vi "Close Subpanel UI Reference.vi"(0 "Plugin in":refnum<class "Generic Plugin.lvclass">, 1 "error in (no error)":errorcluster) -> (2 "Plugin out":refnum<class "Generic Plugin.lvclass">, 4 "error out":errorcluster)   [LabVIEW 2020, in "RxnRover.lvlib" / "Generic Plugin.lvclass"]
doc: "Closes the subpanel UI VI reference and clears the corresponding class attribute."
uses:
  Generic Plugin.lvclass
  Generic Plugin.lvclass/Generic Plugin.ctl
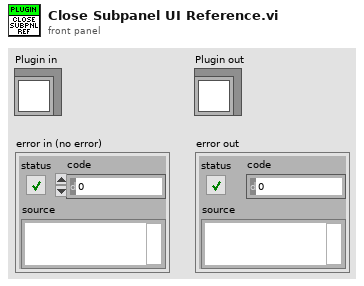
[diagram p1: front panel]
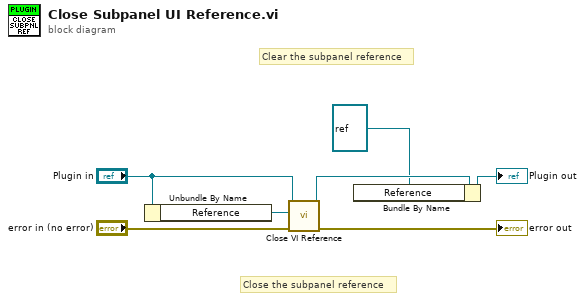
[diagram p0: block diagram]
diagram:
  # "Close the subpanel reference"
  # "Clear the subpanel reference"
  n1 = Unbundle By Name("Plugin in") -> ("Reference"=w3:refnum<vi>)
  n2 = call "Close VI Reference.vi"("error in (no error)"="error in (no error)", "VI Refnum"=w3, "Plugin Server in"="Plugin in") -> ("error out"=→"error out":errorcluster, "Plugin Server out"=w5:refnum<class "Generic Plugin.lvclass">)  [unwired: 6 in, 1 out]
  n3 = Bundle By Name(cluster=w5, "Reference"=refnum<vi> refnum ("Subpanel.Reference")) -> (→"Plugin out":refnum<class "Generic Plugin.lvclass">)
